vi "Get Group Configuration.vi"(8 "error in (no error)":errorcluster, 11 "Component Configuration in":refnum<class "Component Configurations.lvclass">) -> (0 "error out":errorcluster, 1 "Tx Group Configuration":refnum<class "Configuration.lvclass">, 2 "Rx Group Configuration":refnum<class "Configuration.lvclass">, 3 "Component Configuration out":refnum<class "Component Configurations.lvclass">)   [LabVIEW 2019, in "DSF Core.lvlib" / "Component Configurations.lvclass"]
uses:
  Component Configurations.lvclass
  Configuration/Configuration.lvclass
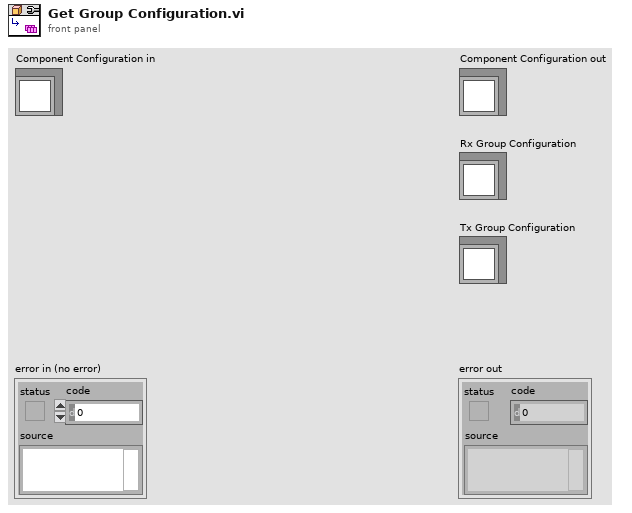
[diagram p1: front panel]
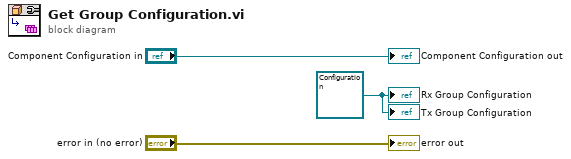
[diagram p0: block diagram]
diagram:
  w1 = refnum<class "Configuration.lvclass"> refnum ("Rx Group Configuration")
  "error out" <- "error in (no error)"
  "Component Configuration out" <- "Component Configuration in"
  "Rx Group Configuration" <- w1
  "Tx Group Configuration" <- w1
